vi "WriteSV.vi"(8 "error in (no error)":errorcluster, 10 "DBL Data":dbl, 11 "shared variable refnum in":refnum<k21>) -> (0 "error out":errorcluster)   [LabVIEW 2016, in "Shared Variable Interface.lvlib" / "Bool.lvlib"]
uses:
  Bool.lvlib
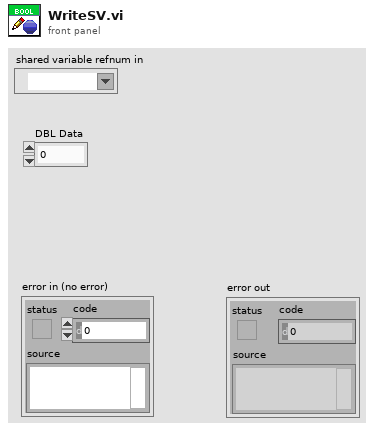
[diagram p1: front panel]
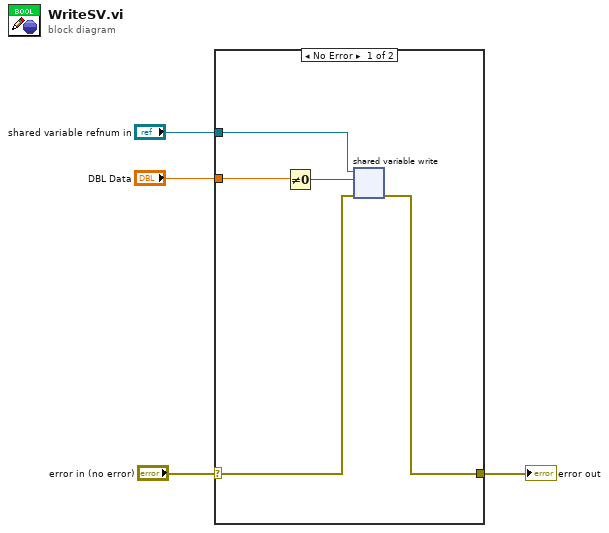
[diagram p0: block diagram]
diagram:
  n1 = case shown="No Error" "error in (no error)" {
    selector: "error in (no error)" -> [w6 w10]
    tunnel: [w9 w10] -> w4
    tunnel: "DBL Data" -> [w7 _]
    tunnel: "shared variable refnum in" -> [w5 _]
    frame No Error {
      n2 = Not Equal To 0?(x=w7) -> (x != 0?=w8:bool)
      n3 = shared-variable-write(w5, w6, w8) -> (w9:errorcluster)  [unwired: 1 out]
    }
    frame Error {
    }
  }
  "error out" <- w4
